vi "ke37xx Get Measurement Buffer Reading Count.vi"(0 "VISA Resource Name":refnum<visa-resource-name>, 7 "Buffer Name":string, 11 "error in (no error)":errorcluster) -> (4 "VISA Resource Name Out":refnum<visa-resource-name>, 8 "Reading Count":u32, 15 "error out":errorcluster)   [LabVIEW 2009, in "Keithley 3700 Series.lvlib"]
doc: "This VI queries the instrument for the number of readings currently stored in the specified reading buffer."
uses:
  <instrlib>/Keithley 3706/Keithley 3700 Series.lvlib
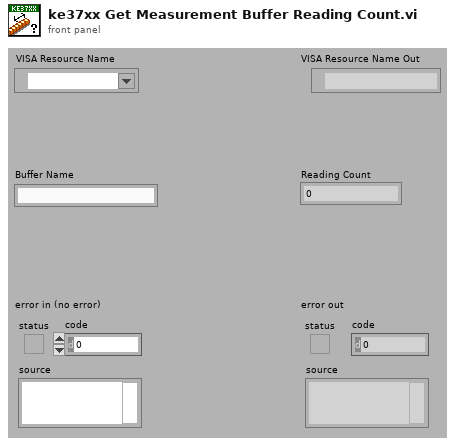
[diagram p1: front panel]
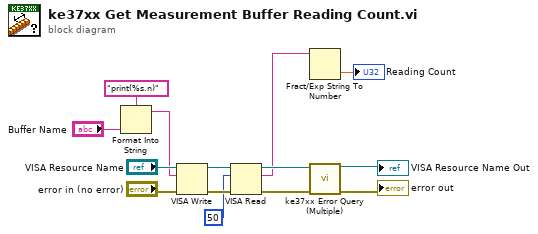
[diagram p0: block diagram]
diagram:
  n1 = Format Into String(format string="print(%s.n)", "Buffer Name") -> (resulting string=w2:string)  [unwired: 2 in, 1 out]
  n2 = VISA Write(VISA resource name="VISA Resource Name", write buffer=w2, error in (no error)="error in (no error)") -> (VISA resource name out=w8:refnum<visa-resource-name>, error out=w6:errorcluster)  [unwired: 1 out]
  n3 = VISA Read(VISA resource name=w8, byte count=u32 50, error in (no error)=w6) -> (VISA resource name out=w7:refnum<visa-resource-name>, read buffer=w4:string, error out=w5:errorcluster)  [unwired: 1 out]
  n4 = Fract/Exp String To Number(string=w4) -> (number=→"Reading Count":dbl)  [unwired: 4 out]
  n5 = call <instrlib>:"ke37xx Error Query (Multiple).vi"("VISA resource name"=w7, "error in (no error)"=w5) -> ("VISA resource name out"=→"VISA Resource Name Out":refnum<visa-resource-name>, "error out"=→"error out":errorcluster)  [unwired: 12 out]
